vi "Drop Database.vi"(0 "InfluxDB in":refnum<class "Client.lvclass">, 5 "Database name":string, 11 "error in (no error)":errorcluster) -> (4 "InfluxDB out":refnum<class "Client.lvclass">, 15 "error out":errorcluster)   [LabVIEW 2018, in "InfluxDB Client.lvlib" / "Client.lvclass"]
doc: "Creates a database."
uses:
  Client.lvclass
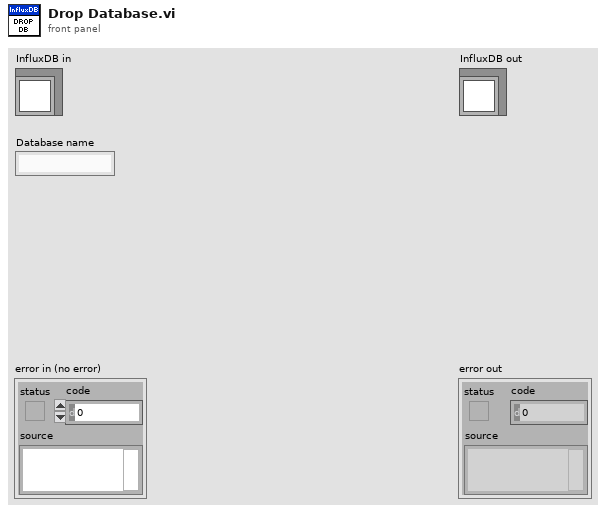
[diagram p1: front panel]
types:
  T1 = typedef "Dictionary Object RefNum__ogtk.ctl" = refnum<k1>
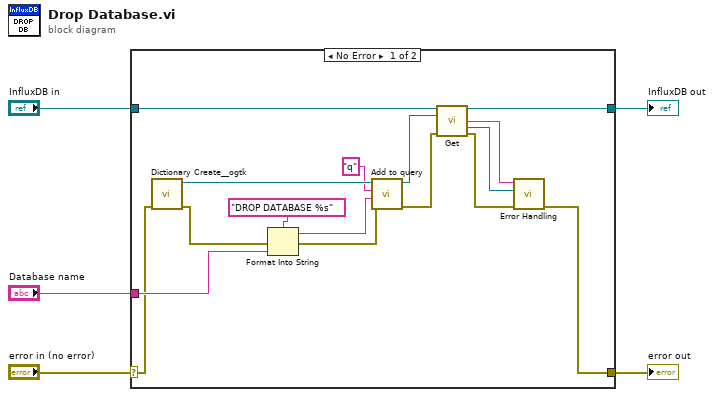
[diagram p0: block diagram]
diagram:
  n1 = case shown="No Error" "error in (no error)" {
    selector: "error in (no error)" -> [w11 w23]
    tunnel: [w6 w23] -> w4
    tunnel: [w20 w22] -> w2
    tunnel: "InfluxDB in" -> [w21 w22]
    tunnel: "Database name" -> [w16 _]
    frame No Error {
      n2 = call <userlib>:"Dictionary Create__ogtk.vi"("error in (no error)"=w11) -> ("error out"=w10:errorcluster, "dictionary out"=w19:T1)  [unwired: 9 in]
      n3 = Format Into String(format string="DROP DATABASE %s" ("Username"), error in=w10, w16) -> (resulting string=w14:string, error out=w13:errorcluster)  [unwired: 1 in]
      n4 = call "Add to query.vi"("error in (no error)"=w13, "Value"=w14, "Parameter"="q" ("String"), "Query in"=w19) -> ("error out"=w12:errorcluster, "Query out"=w17:T1)  [unwired: 6 in]
      n5 = call "Get.vi"("InfluxDB Client in"=w21, "Query"=w17, "error in (no error)"=w12) -> ("InfluxDB Client out"=w20:refnum<class "Client.lvclass">, "Status code"=w9:string, "Headers"=w8:T1, "error out"=w7:errorcluster)  [unwired: 8 in, 1 out]
      n6 = call "Error Handling.vi"("error in (no error)"=w7, "HTTP headers"=w8, "HTTP status code"=w9) -> ("error out"=w6:errorcluster)  [unwired: 8 in]
    }
    frame Error {
    }
  }
  "error out" <- w4
  "InfluxDB out" <- w2
